vi "device-insert-info.vi"(10 "info":T2, 11 "device":T1) -> (3 "device output":T1)   [LabVIEW 2019]
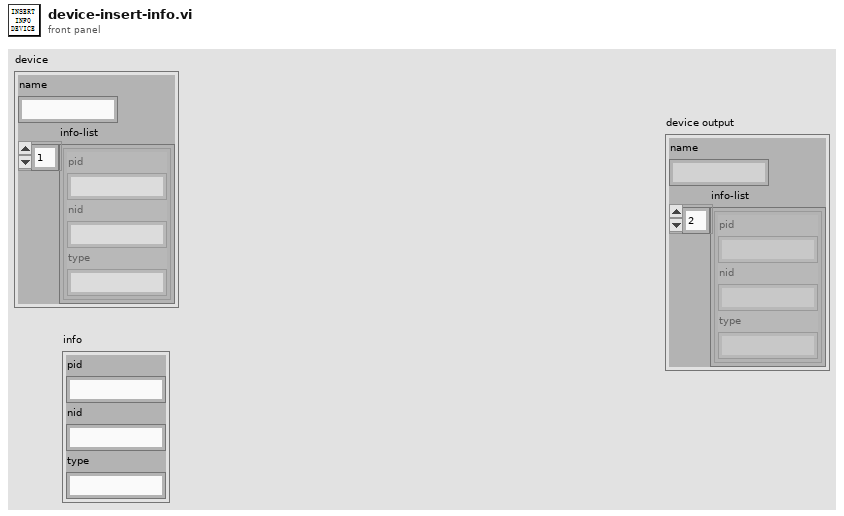
[diagram p1: front panel]
types:
  T1 = cluster{"name":string, "info-list":cluster{"pid":string, "nid":string, "type":string}[]}
  T2 = cluster{"pid":string, "nid":string, "type":string}
  T3 = cluster{"pid":string, "nid":string, "type":string}[]
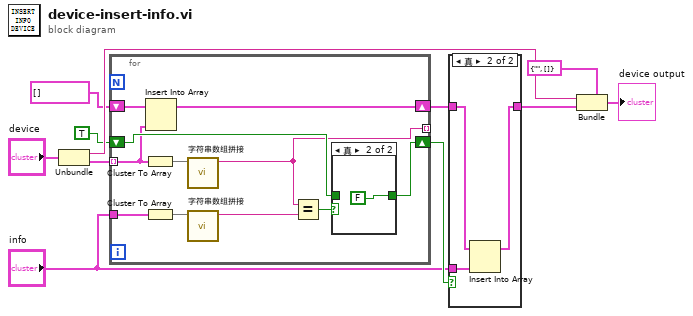
[diagram p0: block diagram]
diagram:
  n1 = Unbundle("device") -> ("name"=w7:string, "info-list"=w10:T3)
  n2 = for {
    tunnel: w10 -> [w15] mode=indexing
    tunnel: "info" -> [w22]
    shift-right: [w17] -> w4
    shift-left: TRUE -> [w16]
    shift-right: [w12] -> w3
    shift-left: T3 [] -> [w14]
    tunnel: [w13] -> _ mode=indexing
    n3 = Cluster To Array(cluster=w15) -> (array=w21:string[])
    n4 = Cluster To Array(cluster=w22) -> (array=w20:string[])
    n5 = Insert Into Array(array=w14, new element=w15) -> (w12:T3)  [unwired: 1 in]
    n6 = call "字符串数组拼接.vi"("数组"=w21) -> ("字符串"=w13:string)  [unwired: 10 in]
    n7 = call "字符串数组拼接.vi"("数组"=w20) -> ("字符串"=w19:string)  [unwired: 10 in]
    n8 = Equal?(x=w13, y=w19) -> (x = y?=w18:bool)
    n9 = case shown="真" w18 {
      tunnel: [w23 FALSE] -> w17
      tunnel: w16 -> [w23 _]
      frame False {
      }
      frame True {
      }
    }
  }
  n10 = case shown="真" w4 {
    tunnel: w3 -> [w25 w28]
    tunnel: "info" -> [_ w27]
    tunnel: [w25 w26] -> w1
    frame False {
    }
    frame True {
      n11 = Insert Into Array(array=w28, new element=w27) -> (w26:T3)  [unwired: 1 in]
    }
  }
  n12 = Bundle(cluster=T1 {"name"="", "info-list"=[]} ("device output"), "name"=w7, "info-list"=w1) -> (→"device output":T1)
